vi "photocelltest.vi"() -> ()   [LabVIEW 2016]
uses:
  <vilib>/LabVIEW Interface for Arduino/LabVIEW Interface for Arduino.lvlib
panel:
  out "Voltage 6":dbl(knob) scale=0.0..5.0
  out "Voltage 5":dbl(knob) scale=0.0..5.0
  out "Voltage 4":dbl(knob) scale=0.0..5.0
  out "Voltage 3":dbl(knob) scale=0.0..5.0
  out "Voltage 2":dbl(knob) scale=0.0..5.0
  out "Voltage":dbl(knob) scale=0.0..5.0
  in  "stop":bool
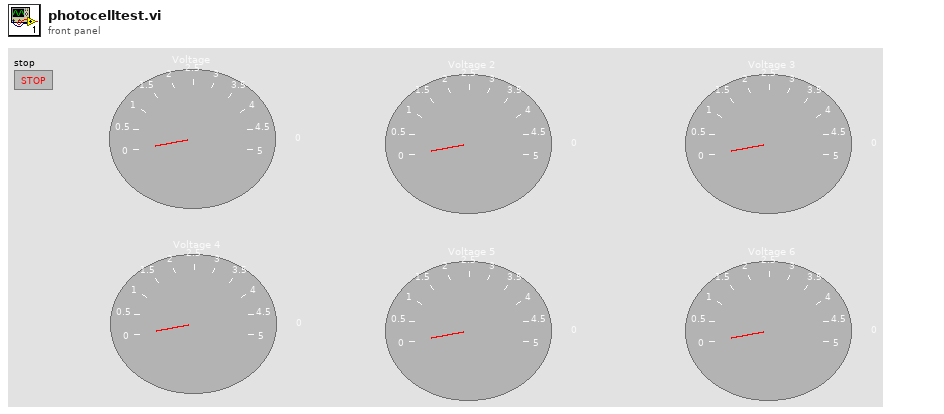
[diagram p1: front panel]
types:
  T1 = typedef "LabVIEW Interface for Arduino.lvlib/Arduino Resource.ctl" = cluster{"VISA resource":refnum<visa-resource-name>, "Board Type":T2, "Connection Type":enum8{"USB / Serial"}, "Bytes Per Packet (15)":u8}
  T2 = typedef "LabVIEW Interface for Arduino.lvlib/Board Type.ctl" = enum16{"Uno", "Dimuelanove w/Atmega 328", "Mega 2560"}
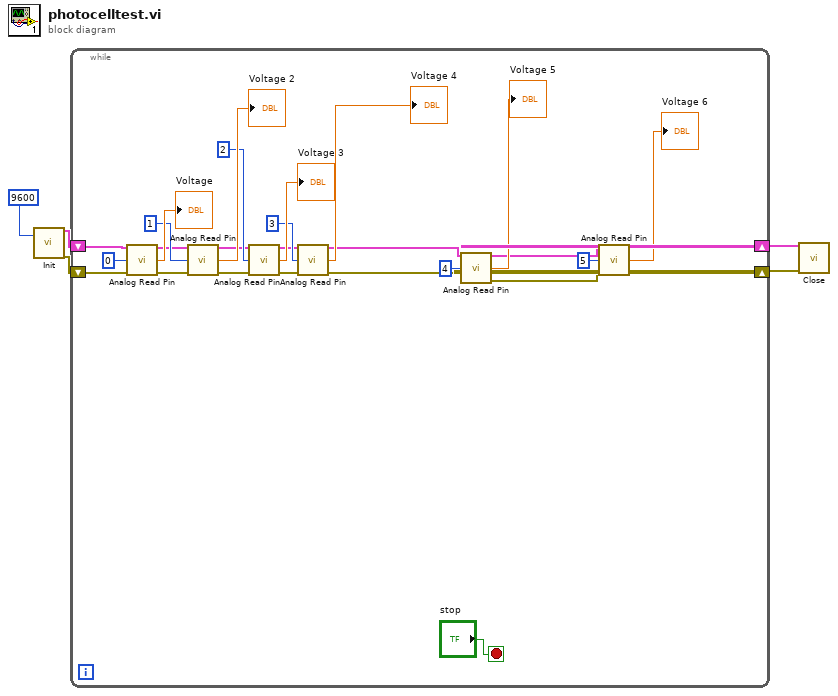
[diagram p0: block diagram]
diagram:
  n1 = call <vilib>:"Init.vi"("Baud Rate (115200)"=u32 9600) -> ("Arduino Resource"=w5:T1, "error out"=w3:errorcluster)  [unwired: 17 in]
  n2 = while {
    shift-right: [w8] -> w4
    shift-left: w5 -> [w25]
    shift-right: [w6] -> w2
    shift-left: w3 -> [w24]
    stop <- "stop" stop-if-true
    n3 = call <vilib>:"Analog Read Pin.vi"("Arduino Resource"=w25, "Analog Input Pin (0)"=u8 0, "error in"=w24) -> ("Arduino Resource"=w22:T1, "Voltage"=→"Voltage":dbl, "error out"=w23:errorcluster)  [unwired: 10 in]
    n4 = call <vilib>:"Analog Read Pin.vi"("Arduino Resource"=w22, "Analog Input Pin (0)"=u8 1, "error in"=w23) -> ("Arduino Resource"=w21:T1, "Voltage"=→"Voltage 2":dbl, "error out"=w20:errorcluster)  [unwired: 10 in]
    n5 = call <vilib>:"Analog Read Pin.vi"("Arduino Resource"=w21, "Analog Input Pin (0)"=u8 2, "error in"=w20) -> ("Arduino Resource"=w17:T1, "Voltage"=→"Voltage 3":dbl, "error out"=w16:errorcluster)  [unwired: 10 in]
    n6 = call <vilib>:"Analog Read Pin.vi"("Arduino Resource"=w17, "Analog Input Pin (0)"=u8 3, "error in"=w16) -> ("Arduino Resource"=w13:T1, "Voltage"=→"Voltage 4":dbl, "error out"=w12:errorcluster)  [unwired: 10 in]
    n7 = call <vilib>:"Analog Read Pin.vi"("Arduino Resource"=w13, "Analog Input Pin (0)"=u8 4, "error in"=w12) -> ("Arduino Resource"=w9:T1, "Voltage"=→"Voltage 5":dbl, "error out"=w7:errorcluster)  [unwired: 10 in]
    n8 = call <vilib>:"Analog Read Pin.vi"("Arduino Resource"=w9, "Analog Input Pin (0)"=u8 5, "error in"=w7) -> ("Arduino Resource"=w8:T1, "Voltage"=→"Voltage 6":dbl, "error out"=w6:errorcluster)  [unwired: 10 in]
  }
  n9 = call <vilib>:"Close.vi"("Arduino Resource"=w4, "error in"=w2) -> ()  [unwired: 13 in, 1 out]
